vi "Make clump.vi"(10 "Veristand Type":T3, 11 "Channels":T1[](array[typedef])) -> (3 "Cluster out":T6)   [LabVIEW 2015]
uses:
  <vilib>/NI Veristand/Custom Device API/Custom Device Channel Type.ctl
  <vilib>/NI VeriStand/Custom Device API/Custom Device API.lvlib
  System Explorer/SubVIs/Modbus Type.ctl
  Shared/Modbus Master Shared.lvlib
  Shared/Controls/Data Model/DataType.ctl
  Shared/Controls/Data Model/Mapping.ctl
  Form Clump.ctl
  Shared/Controls/Data Model/Channel.ctl
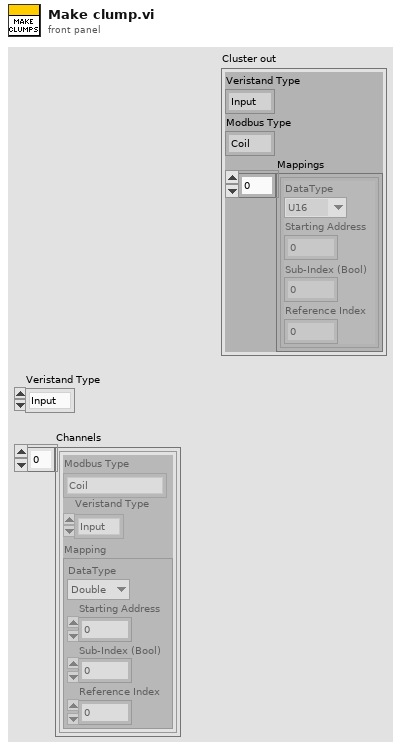
[diagram p1: front panel]
types:
  T1 = typedef "Modbus Master Shared.lvlib/Channel.ctl" = cluster{"Modbus Type":T2, "Veristand Type":T3, "Mapping":T4}
  T2 = typedef "Modbus Master Shared.lvlib/Modbus Type.ctl" = enum16{"Coil", "Discrete Input", "Holding Register", "Input Register"}
  T3 = typedef "Custom Device API.lvlib/Custom Device Channel Type.ctl" = enum16{"Input", "Output"}
  T4 = typedef "Modbus Master Shared.lvlib/Mapping.ctl" = cluster{"DataType":T5, "Starting Address":u16, "Sub-Index (Bool)":u16, "Reference Index":u16}
  T5 = typedef "Modbus Master Shared.lvlib/DataType.ctl" = enum16{"Double", "Single", "I64", "I32", "I16", "I8", "U64", "U32", "U16", "U8", "Boolean"}
  T6 = typedef "Modbus Master Shared.lvlib/Form Clump.ctl" = cluster{"Veristand Type":T3, "Modbus Type":T2, "Mappings":T4[]}
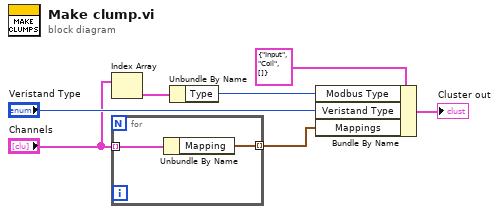
[diagram p0: block diagram]
diagram:
  n1 = Index Array(array="Channels") -> (element=w2:T1)  [unwired: 1 in]
  n2 = for {
    tunnel: "Channels" -> [w9] mode=indexing
    tunnel: [w8] -> w4 mode=indexing
    n3 = Unbundle By Name(w9) -> ("Mapping"=w8:T4)
  }
  n4 = Unbundle By Name(w2) -> ("Type"=w5:T2)
  n5 = Bundle By Name(cluster=T6 {"Veristand Type"=enum."Input", "Modbus Type"=enum."Coil", "Mappings"=[]} ("Cluster in"), "Modbus Type"=w5, "Veristand Type"="Veristand Type", "Mappings"=w4) -> (→"Cluster out":T6)
